vi "Interpolate 1 Unit Steps.vi"(11 "String In":string) -> (3 "String Out":string)   [LabVIEW 2019]
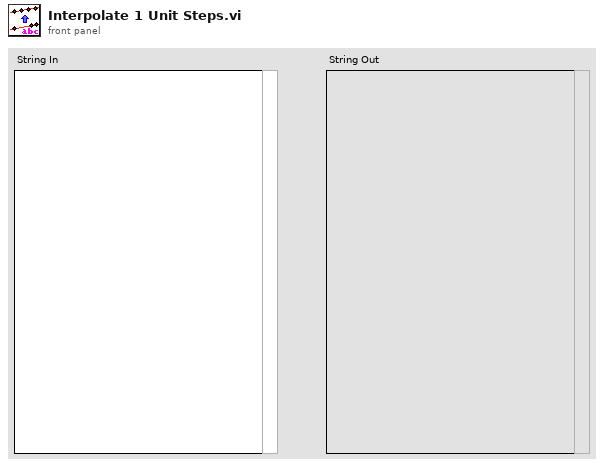
[diagram p1: front panel]
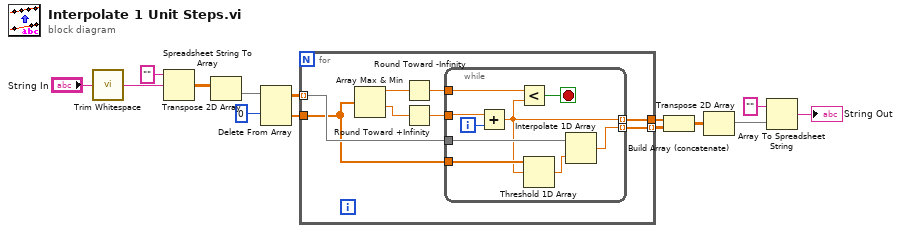
[diagram p0: block diagram]
diagram:
  n1 = call <vilib>:"Trim Whitespace.vi"("string"="String In") -> ("trimmed string"=w3:string)  [unwired: 1 in]
  n2 = Spreadsheet String To Array(format string="", spreadsheet string=w3) -> (array=w12:dbl[][])  [unwired: 2 in]
  n3 = Transpose 2D Array(2D array=w12) -> (transposed array=w2:dbl[][])
  n4 = Delete From Array(array=w2, index (row)=0 ("index (col)")) -> (deleted portion=w10:dbl[], array with subset deleted=w11:dbl[][])  [unwired: 2 in]
  n5 = for {
    tunnel: w11 -> [w18] mode=indexing
    tunnel: w10 -> [w17]
    tunnel: [w16] -> w9
    tunnel: [w15] -> w8 mode=indexing
    n6 = Array Max & Min(array=w17) -> (max value=w21:dbl, min value=w22:dbl)  [unwired: 2 out]
    n7 = Round Toward -Infinity(1:w21) -> (0:w19:dbl)
    n8 = Round Toward +Infinity(x=w22) -> (ceil(x): smallest int >= x=w20:dbl)
    n9 = while {
      tunnel: w20 -> [w31]
      tunnel: w19 -> [w29]
      tunnel: w18 -> [w27]
      tunnel: w17 -> [w26]
      tunnel: [w24] -> w15 mode=indexing
      tunnel: [w23] -> w16 mode=indexing
      i -> [w30]
      stop <- w28 stop-if-true
      n10 = Add(x=w31, y=w30) -> (x+y=w23:dbl)
      n11 = Less?(x=w29, y=w23) -> (x < y?=w28:bool)
      n12 = Threshold 1D Array(2:w23, 3:w26) -> (0:w25:dbl)  [unwired: 1 in]
      n13 = Interpolate 1D Array(1:w25, 2:w27) -> (0:w24:dbl)
    }
  }
  n14 = Build Array (concatenate)(w9, w8) -> (w7:dbl[][])
  n15 = Transpose 2D Array(2D array=w7) -> (transposed array=w6:dbl[][])
  n16 = Array To Spreadsheet String(array=w6, 3:"" ("format string")) -> (spreadsheet string=→"String Out":string)  [unwired: 1 in]
